vi "Day 1-2.vi"() -> ()   [LabVIEW 2019, in "Day 1.lvlib"]
uses:
  Day 1.lvlib
panel:
  out "Result":i32
  out "Array":i32[](array[numeric])
  in  "String":string="124\n125\n127\n128\n132\n140\n142\n103\n102\n110\n101\n107\n109\n113\n119\n120\n122\n124\n125\n121\n119\n139\n159\n164\n165\n177\n190\n181\n182\n171\n192\n185\n184\n186\n183\n203\n204\n209\n210\n214\n215\n213\n235\n257\n271\n278\n279\n284\n286\n289\n290\n287\n291\n297\n287\n290\n273\n280\n284\n288\n289\n294\n310\n324\n319\n320\n324\n325\n327\n328\n326\n328\n300\n301\n302\n306\n308\n315\n349\n364\n365\n367\n369\n376\n384\n386\n378\n382\n396\n427\n435\n434\n437\n424\n432\n443\n453\n451\n453\n440\n446\n447\n448\n449\n454\n462\n463\n448\n447\n448\n460\n468\n469\n470\n473\n479\n480\n481\n488\n498\n499\n502\n504\n510\n513\n507\n506\n504\n507\n518\n520\n519\n515\n520\n536\n534\n535\n537\n554\n555\n556\n558\n554\n566\n558\n542\n545\n552\n556\n563\n..."
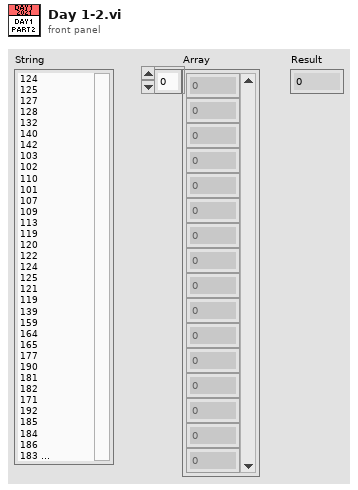
[diagram p1: front panel]
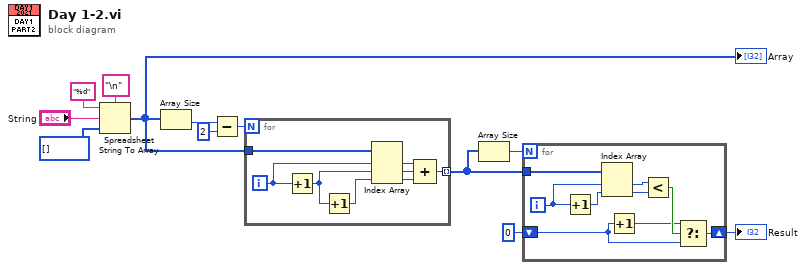
[diagram p0: block diagram]
diagram:
  n1 = Spreadsheet String To Array(delimiter (Tab)="\n", format string="%d", spreadsheet string="String", array type (2D Dbl)=i32[] []) -> (array=w1:i32[])
  "Array" <- w1
  n2 = Array Size(array=w1) -> (size(s)=w9:i32)
  n3 = Subtract(x=w9, y=2) -> (x-y=w7:i32)
  n4 = for {
    N: w7 -> [_]
    tunnel: w1 -> [w20]
    tunnel: [w13] -> w6 mode=indexing
    i -> [w19]
    n5 = Increment(x=w19) -> (x+1=w17:i32)
    n6 = Increment(x=w17) -> (x+1=w18:i32)
    n7 = Index Array(array=w20, index #1=w19, index #2=w17, index #3=w18) -> (element #1=w16:i32, element #2=w15:i32, element #3=w14:i32)
    n8 = Compound Arithmetic op=ADD(w16, w15, w14) -> (w13:i32)
  }
  n9 = Array Size(array=w6) -> (size(s)=w12:i32)
  n10 = for {
    N: w12 -> [_]
    tunnel: w6 -> [w29]
    shift-right: [w21] -> w11
    shift-left: 0 -> [w22]
    i -> [w28]
    n11 = Increment(x=w28) -> (x+1=w27:i32)
    n12 = Index Array(array=w29, index #1=w28, index #2=w27) -> (element #1=w26:i32, element #2=w25:i32)
    n13 = Increment(x=w22) -> (x+1=w23:i32)
    n14 = Less?(x=w26, y=w25) -> (x < y?=w24:bool)
    n15 = Select(t=w23, s=w24, f=w22) -> (s? t:f=w21:i32)
  }
  "Result" <- w11
